vi "Init Talon Gripper Motors With CVS File.vi"(1 "Robot ID":string="981") -> (0 "RobotDriveDevRef":T1={"DevStatus"={"status"=FALSE, "code"=0, "source"=""}, "Motors[]"=[], "Square Inputs"=FALSE, "Max Output"=1.0})   [LabVIEW 2017]
uses:
  <vilib>/Rock Robotics/WPI/RobotDrive/WPI_RobotDriveDevRef.ctl
  <vilib>/Rock Robotics/WPI/MotorControl/WPI_MotorControlDeviceRef.ctl
  <vilib>/Rock Robotics/WPI/MotorControl/WPI_MotorControlType.ctl
  <vilib>/Rock Robotics/SystemInterfaces/DIO/FPGA_DIOPWMChannel.ctl
  <vilib>/Rock Robotics/WPI/PWM/WPI_PWMDeadband.ctl
  <vilib>/Rock Robotics/SystemInterfaces/DIO/FPGA_DIOChannel.ctl
  <vilib>/Rock Robotics/WPI/RobotDrive/WPI_RobotDriveOpen2MotorWithExistingMotors.vi
panel:
  out "Gripper Right":i32
  out "Gripper Left":i32
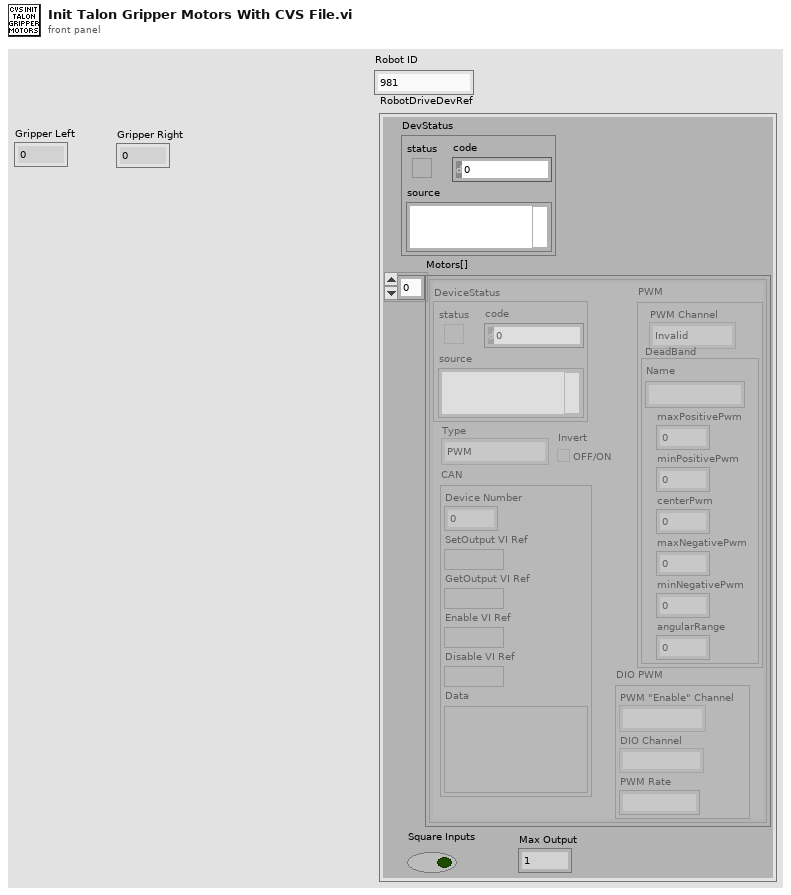
[diagram p1: front panel]
types:
  T1 = typedef "WPI_RobotDriveDevRef.ctl" = cluster{"DevStatus":errorcluster, "Motors[]":T2[], "Square Inputs":bool, "Max Output":dbl}
  T2 = typedef "WPI_MotorControlDeviceRef.ctl" = cluster{"DeviceStatus":errorcluster, "Type":T3, "PWM":cluster{"PWM Channel":T4, "DeadBand":T5}, "CAN":cluster{"Device Number":u8, "SetOutput VI Ref":variant, "GetOutput VI Ref":variant, "Enable VI Ref":variant, "Disable VI Ref":variant, "Data":variant}, "Invert":bool, "DIO PWM":cluster{"PWM \"Enable\" Channel":T4, "DIOChannel":T6, "PWM Rate":dbl}}
  T3 = typedef "WPI_MotorControlType.ctl" = enum16{"PWM", "CAN", "DIO PWM"}
  T4 = typedef "FPGA_DIOPWMChannel.ctl" = enum8{"PWM 0", "PWM 1", "PWM 2", "PWM 3", "PWM 4", "PWM 5", "PWM 6", "PWM 7", "PWM 8", "PWM 9", "PWM MXP 0", "PWM MXP 1", "PWM MXP 2", "PWM MXP 3", "PWM MXP 4", "PWM MXP 5", "PWM MXP 6", "PWM MXP 7", "PWM MXP 8", "PWM MXP 9", "Invalid"}
  T5 = typedef "WPI_PWMDeadband.ctl" = cluster{"Name":string, "maxPositivePwm":i32, "minPositivePwm":i32, "centerPwm":i32, "maxNegativePwm":i32, "minNegativePwm":i32, "angularRange":u16}
  T6 = typedef "FPGA_DIOChannel.ctl" = enum8{"DIO 0", "DIO 1", "DIO 2", "DIO 3", "DIO 4", "DIO 5", "DIO 6", "DIO 7", "DIO 8", "DIO 9", "DIO MXP 0", "DIO MXP 1", "DIO MXP 2", "DIO MXP 3", "DIO MXP 4", "DIO MXP 5", "DIO MXP 6", "DIO MXP 7", "DIO MXP 8", "DIO MXP 9", "DIO MXP 10", "DIO MXP 11", "DIO MXP 12", "DIO MXP 13", "DIO MXP 14", "DIO MXP 15", "SPI Port CS1", "SPI Port CS2", "SPI Port CS3", "SPI Port MISO", "SPI Port MOSI", "Invalid"}
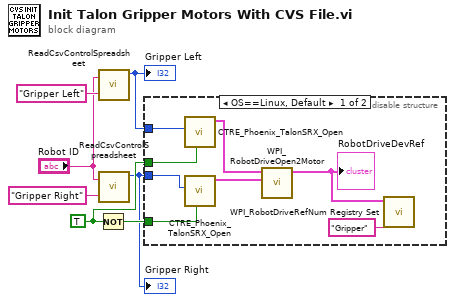
[diagram p0: block diagram]
diagram:
  w4 = TRUE
  n1 = Not(x=w4) -> (.not. x?=w3:bool)
  n2 = call "ReadCsvControlSpreadsheet.vi"("Robot ID"="Robot ID", "Motor ID"="Gripper Left") -> ("Can Bus ID"=w2:u8)  [unwired: 3 out]
  "Gripper Left" <- w2
  n3 = call "ReadCsvControlSpreadsheet.vi"("Robot ID"="Robot ID", "Motor ID"="Gripper Right") -> ("Can Bus ID"=w1:u8)  [unwired: 3 out]
  "Gripper Right" <- w1
  n4 = disable-structure shown="OS==Linux, Default" {
    disable-tunnel: w4 -> [w15 _]
    disable-tunnel: w3 -> [w14 _]
    disable-tunnel: w2 -> [w11 _]
    disable-tunnel: w1 -> [w10 _]
    frame condition #0 (active) {
      n5 = call "CTRE_Phoenix_TalonSRX_Open.vi"("Invert"=w15, "Device Number"=w11) -> ("CAN Talon SRX Ref"=w13:T2)  [unwired: 8 in, 1 out]
      n6 = call "CTRE_Phoenix_TalonSRX_Open.vi"("Invert"=w14, "Device Number"=w10) -> ("CAN Talon SRX Ref"=w12:T2)  [unwired: 8 in, 1 out]
      n7 = call-poly <vilib>:"WPI_RobotDriveOpen2Motor.vi"("Right Motor Dev Ref"=w12, "Left Motor Dev Ref"=w13) -> ("RobotDriveDevRef"=w9:T1)  [unwired: 8 in, 1 out]
      "RobotDriveDevRef" <- w9
      n8 = call <vilib>:"WPI_RobotDriveRefNum Registry Set.vi"("refnum name"="Gripper", "RobotDriveDevRef"=w9) -> ()  [unwired: 8 in, 2 out]
    }
    frame condition #1 {
    }
  }
